vi "Scan.vi"(8 "error in":errorcluster, 11 "variant in":variant) -> (0 "error out":errorcluster, 3 "variant out":variant, 4 "Scanning":bool)   [LabVIEW 2013]
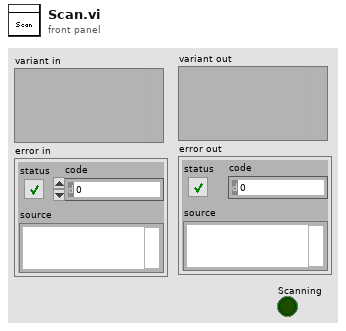
[diagram p1: front panel]
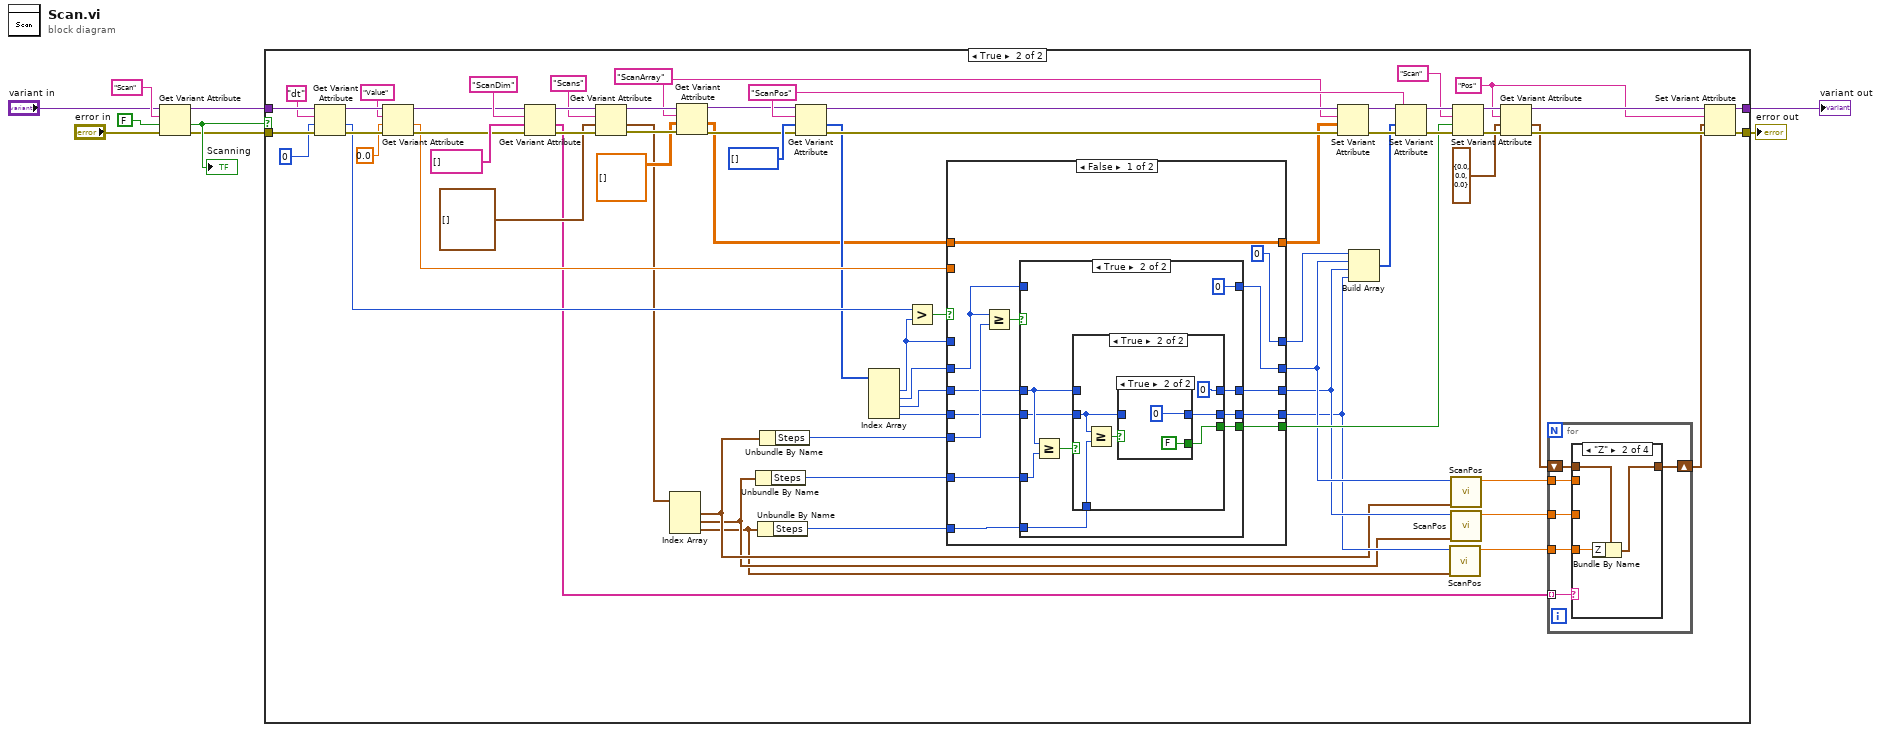
[diagram p0: block diagram]
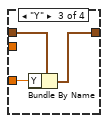
[diagram p4: hidden frame]
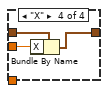
[diagram p5: hidden frame]
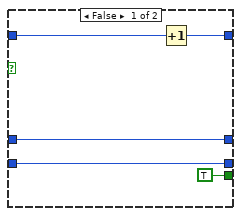
[diagram p6: hidden frame]
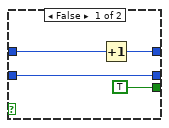
[diagram p7: hidden frame]
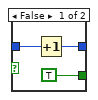
[diagram p8: hidden frame]
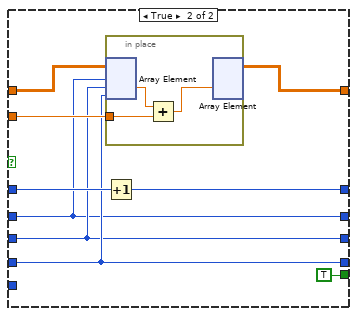
[diagram p9: hidden frame]
diagram:
  n1 = Get Variant Attribute(Variant="variant in", name="Scan", default value (empty Variant)=FALSE, error in="error in") -> (duplicate Variant=w7:variant, value=w9:bool, error out=w8:errorcluster)  [unwired: 1 out]
  "Scanning" <- w9
  n2 = case shown="True" w9 {
    tunnel: [w11 w35] -> w2
    tunnel: w7 -> [w11 w74]
    tunnel: [w10 w34] -> w1
    tunnel: w8 -> [w10 w73]
    frame False {
    }
    frame True {
      w28 = "Pos" ("name")
      w46 = "ScanArray" ("name")
      w75 = "ScanPos" ("name")
      n3 = Get Variant Attribute(Variant=w74, name="dt", default value (empty Variant)=0, error in=w73) -> (duplicate Variant=w67:variant, value=w61:i32, error out=w64:errorcluster)  [unwired: 1 out]
      n4 = Get Variant Attribute(Variant=w67, name="Value", default value (empty Variant)=0.0, error in=w64) -> (duplicate Variant=w66:variant, value=w51:dbl, error out=w65:errorcluster)  [unwired: 1 out]
      n5 = Get Variant Attribute(Variant=w66, name="ScanDim", default value (empty Variant)=string[] [], error in=w65) -> (duplicate Variant=w79:variant, value=w27:string[], error out=w78:errorcluster)  [unwired: 1 out]
      n6 = Get Variant Attribute(Variant=w79, name="Scans", default value (empty Variant)=cluster{"Start":dbl, "Stop":dbl, "Steps":u32}[] [], error in=w78) -> (duplicate Variant=w59:variant, value=w44:cluster{"Start":dbl, "Stop":dbl, "Steps":u32}[], error out=w56:errorcluster)  [unwired: 1 out]
      n7 = Index Array(array=w44) -> (element #1=w17:cluster{"Start":dbl, "Stop":dbl, "Steps":u32}, element #2=w16:cluster{"Start":dbl, "Stop":dbl, "Steps":u32}, element #3=w15:cluster{"Start":dbl, "Stop":dbl, "Steps":u32})  [unwired: 3 in]
      n8 = Get Variant Attribute(Variant=w59, name=w46, default value (empty Variant)=dbl[][][] [] ("initialized array"), error in=w56) -> (duplicate Variant=w58:variant, value=w33:dbl[][][], error out=w57:errorcluster)  [unwired: 1 out]
      n9 = Unbundle By Name(w16) -> ("Steps"=w22:u32)
      n10 = Unbundle By Name(w15) -> ("Steps"=w21:u32)
      n11 = Unbundle By Name(w17) -> ("Steps"=w23:u32)
      n12 = Get Variant Attribute(Variant=w58, name=w75, default value (empty Variant)=i32[] [], error in=w57) -> (duplicate Variant=w50:variant, value=w43:i32[], error out=w49:errorcluster)  [unwired: 1 out]
      n13 = Index Array(array=w43) -> (element #1=w42:i32, element #2=w54:i32, element #3=w53:i32, element #4=w52:i32)  [unwired: 4 in]
      n14 = Greater?(x=w61, y=w42) -> (0:w60:bool)
      n15 = case shown="False" w60 {
        tunnel: w33 -> [w108 w144]
        tunnel: w54 -> [w105 w138]
        tunnel: w53 -> [w104 w139]
        tunnel: w52 -> [w103 w140]
        tunnel: w51 -> [_ w142]
        tunnel: [w108 w143] -> w45
        tunnel: w23 -> [w107 _]
        tunnel: [w102 TRUE] -> w36
        tunnel: [w101 w138] -> w20
        tunnel: [w100 w139] -> w19
        tunnel: [w99 w140] -> w18
        tunnel: [0 w145] -> w41
        tunnel: w42 -> [_ w141]
        tunnel: w22 -> [w97 _]
        tunnel: w21 -> [w96 _]
        frame False {
          n16 = Greater Or Equal?(x=w105, y=w107) -> (x >= y?=w106:bool)
          n17 = case shown="True" w106 {
            tunnel: w105 -> [w110 _]
            tunnel: w104 -> [w113 w121]
            tunnel: w103 -> [w112 w119]
            tunnel: [w109 0] -> w101
            tunnel: [w113 w120] -> w100
            tunnel: [w112 w118] -> w99
            tunnel: [TRUE w117] -> w102
            tunnel: w97 -> [_ w116]
            tunnel: w96 -> [_ w115]
            frame False {
              n18 = Increment(x=w110) -> (x+1=w109:i32)
            }
            frame True {
              n19 = Greater Or Equal?(x=w121, y=w116) -> (x >= y?=w122:bool)
              n20 = case shown="True" w122 {
                tunnel: w121 -> [w123 _]
                tunnel: [w124 0] -> w120
                tunnel: w119 -> [w126 w131]
                tunnel: [w126 w130] -> w118
                tunnel: [TRUE w129] -> w117
                tunnel: w115 -> [_ w128]
                frame False {
                  n21 = Increment(x=w123) -> (x+1=w124:i32)
                }
                frame True {
                  n22 = Greater Or Equal?(x=w131, y=w128) -> (x >= y?=w132:bool)
                  n23 = case shown="True" w132 {
                    tunnel: w131 -> [w133 _]
                    tunnel: [w134 0] -> w130
                    tunnel: [TRUE FALSE] -> w129
                    frame False {
                      n24 = Increment(x=w133) -> (x+1=w134:i32)
                    }
                    frame True {
                    }
                  }
                }
              }
            }
          }
        }
        frame True {
          n25 = in-place {
            in-place-border: w142 -> [w147]
            n26 = in-place-array #1(w144, w138, w139, w140) -> (w149:dbl)
            n27 = Add(x=w149, y=w147) -> (x+y=w148:dbl)
            n28 = in-place-array #1(w148) -> (w143:dbl[][][])  [unwired: 3 out]
          }
          n29 = Increment(x=w141) -> (x+1=w145:i32)
        }
      }
      n30 = Set Variant Attribute(Variant=w50, name=w46, value=w45, error in=w49) -> (Variant out=w48:variant, error out=w47:errorcluster)  [unwired: 1 out]
      n31 = Build Array(w41, w20, w19, w18) -> (w40:i32[])
      n32 = Set Variant Attribute(Variant=w48, name=w75, value=w40, error in=w47) -> (Variant out=w39:variant, error out=w38:errorcluster)  [unwired: 1 out]
      n33 = call "ScanPos.vi"("DimScan"=w15, "ScanPos"=w18) -> ("Pos"=w13:dbl)  [unwired: 9 in]
      n34 = call "ScanPos.vi"("DimScan"=w17, "ScanPos"=w20) -> ("Pos"=w14:dbl)  [unwired: 9 in]
      n35 = call "ScanPos.vi"("DimScan"=w16, "ScanPos"=w19) -> ("Pos"=w12:dbl)  [unwired: 9 in]
      n36 = Set Variant Attribute(Variant=w39, name="Scan", value=w36, error in=w38) -> (Variant out=w31:variant, error out=w32:errorcluster)  [unwired: 1 out]
      n37 = Get Variant Attribute(Variant=w31, name=w28, default value (empty Variant)=cluster{"X":dbl, "Y":dbl, "Z":dbl} {"X"=0.0, "Y"=0.0, "Z"=0.0} ("Relative Position"), error in=w32) -> (duplicate Variant=w30:variant, value=w26:cluster{"X":dbl, "Y":dbl, "Z":dbl}, error out=w29:errorcluster)  [unwired: 1 out]
      n38 = for {
        tunnel: w27 -> [w85] mode=indexing
        shift-right: [w83] -> w24
        shift-left: w26 -> [w84]
        tunnel: w14 -> [w82]
        tunnel: w13 -> [w81]
        tunnel: w12 -> [w80]
        n39 = case shown="\"Z\"" w85 {
          tunnel: w84 -> [w86 w89 w92 w95]
          tunnel: [w86 w88 w91 w94] -> w83
          tunnel: w82 -> [_ _ _ w93]
          tunnel: w81 -> [_ w87 _ _]
          tunnel: w80 -> [_ _ w90 _]
          frame "none", Default {
          }
          frame "Z" {
            n40 = Bundle By Name(cluster=w89, "Z"=w87) -> (w88:cluster{"X":dbl, "Y":dbl, "Z":dbl})
          }
          frame "Y" {
            n41 = Bundle By Name(cluster=w92, "Y"=w90) -> (w91:cluster{"X":dbl, "Y":dbl, "Z":dbl})
          }
          frame "X" {
            n42 = Bundle By Name(cluster=w95, "X"=w93) -> (w94:cluster{"X":dbl, "Y":dbl, "Z":dbl})
          }
        }
      }
      n43 = Set Variant Attribute(Variant=w30, name=w28, value=w24, error in=w29) -> (Variant out=w35:variant, error out=w34:errorcluster)  [unwired: 1 out]
    }
  }
  "variant out" <- w2
  "error out" <- w1
